vi "read event.vi"() -> ()   [LabVIEW 2016]
uses:
  <vilib>/Instr/_visa.llb/Select Event Type.ctl
  <vilib>/Utility/error.llb/DialogType.ctl
  <vilib>/Instr/_visa.llb/VISA Configure Serial Port (Instr).vi
panel:
  out "error out":errorcluster
  out "recv bytes":u32
  out "Waveform Chart":dbl(graph)
  out "read buffer":string
  in  "VISA resource name":refnum<visa-resource-name>
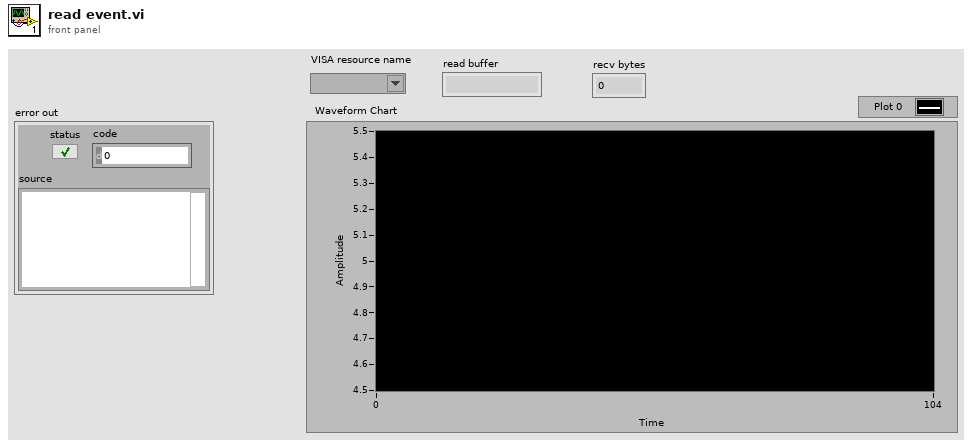
[diagram p1: front panel]
types:
  T1 = typedef "Select Event Type.ctl" = u32
  T2 = typedef "DialogType.ctl" = u16
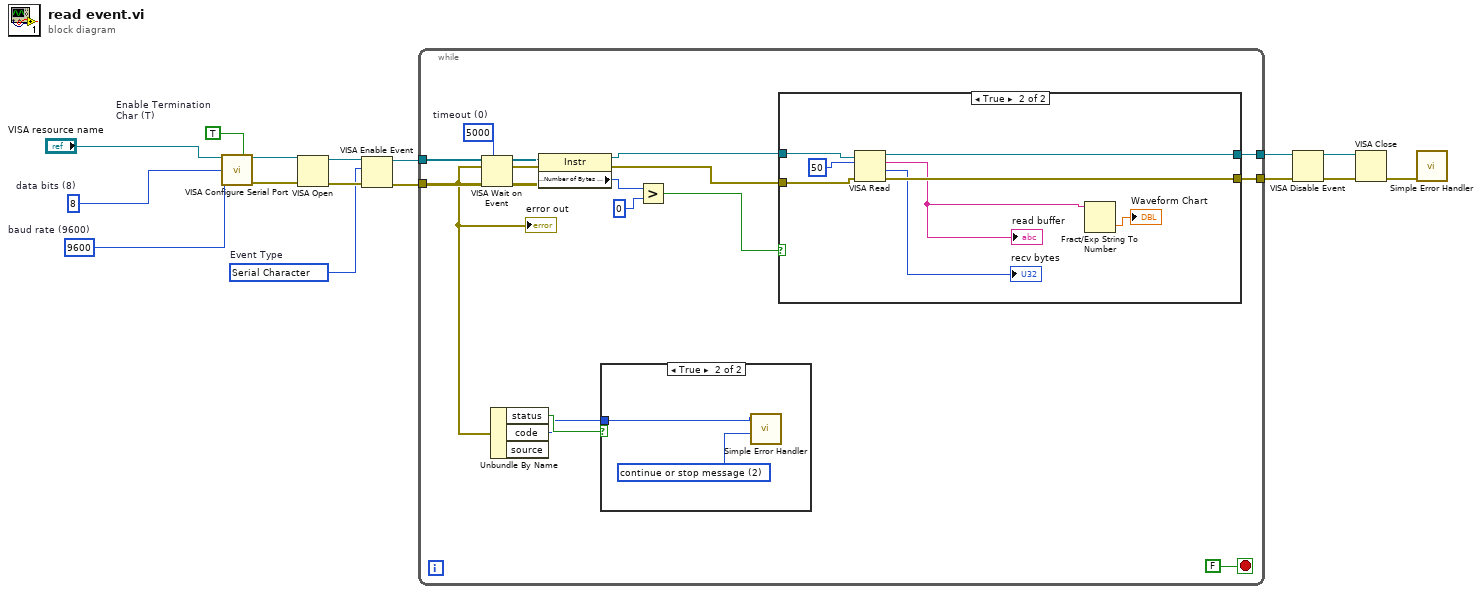
[diagram p0: block diagram]
diagram:
  w4 = u16 8  # data bits (8)
  w5 = TRUE  # Enable Termination Char (T)
  w6 = T1 1073684533 items=["Service Request"=1073684491, "Trigger"=3221168138, "Clear"=1073684493, "VXI Signal"=1073684512, "VXI/VME Interrupt"=3221168161, "VXI/VME Sysfail"=1073684509, "VXI/VME Sysreset"=1073684510, "GPIB CIC"=1073684498, "GPIB Talk"=1073684499, "GPIB Listen"=1073684500, "PXI Interrupt"=1073684514, "Serial Break"=1073684515, "Serial TermChar"=1073684516, "Serial CTS"=1073684521, "Serial DSR"=1073684522, "Serial DCD"=1073684524, "Serial RI"=1073684526, "Serial Character"=1073684533, "USB Interrupt"=1073684535, "All Enabled"=1073709055]  # Event Type
  w15 = u32 9600  # baud rate (9600)
  n1 = call-poly "VISA Configure Serial Port"("VISA resource name"="VISA resource name", "Enable Termination\nChar (T)"=w5, "baud rate (9600)"=w15, "data bits (8)"=w4) -> ("VISA resource name out"=w14:refnum<visa-resource-name>, "error out"=w13:errorcluster)  [unwired: 10 in]
  n2 = VISA Open(error in (no error)=w13, VISA resource name=w14) -> (VISA resource name=w12:refnum<visa-resource-name>, error out=w11:errorcluster)  [unwired: 3 in]
  n3 = VISA Enable Event(8:w11, 10:w6, 11:w12) -> (0:w9:errorcluster, 3:w10:refnum<visa-resource-name>)  [unwired: 1 in]
  n4 = while {
    tunnel: w10 -> [w31]
    tunnel: w9 -> [w30]
    tunnel: [w29] -> w8
    tunnel: [w28] -> w7
    stop <- FALSE stop-if-true
    w21 = u32 5000  # timeout (0)
    n5 = VISA Wait on Event(7:w21, 8:w30, 11:w31) -> (0:w19:errorcluster, 3:w27:refnum<visa-resource-name>)  [unwired: 2 in, 2 out]
    "error out" <- w19
    n6 = Unbundle By Name(w19) -> ("status"=w18:bool, "code"=w17:i32)  [unwired: 1 out]
    n7 = property class="Instr"(reference=w27, error in=w19) -> (reference out=w26:refnum<visa-resource-name>, error out=w22:errorcluster, "Serial Settings:Number of Bytes at Serial Port"=w25:u32)
    n8 = case shown="True" w18 {
      tunnel: w17 -> [_ w33]
      frame False {
      }
      frame True {
        w32 = T2 2 items=["no dialog", "OK message", "continue or stop message", "OK message + warnings", "continue/stop + warnings"] ("type of dialog (OK msg:1)")
        n9 = call <vilib>:"Simple Error Handler.vi"("error code (no error:0)"=w33, "type of dialog (OK msg:1)"=w32) -> ()  [unwired: 3 in, 5 out]
      }
    }
    n10 = Greater?(x=w25, y=u32 0) -> (0:w23:bool)
    n11 = case shown="True" w23 {
      tunnel: [w35 w43] -> w29
      tunnel: [w34 w42] -> w28
      tunnel: w26 -> [w35 w37]
      tunnel: w22 -> [w34 w36]
      frame False {
      }
      frame True {
        n12 = VISA Read(VISA resource name=w37, byte count=u32 50, error in (no error)=w36) -> (VISA resource name out=w43:refnum<visa-resource-name>, read buffer=w40:string, return count=→"recv bytes":u32, error out=w42:errorcluster)
        "read buffer" <- w40
        n13 = Fract/Exp String To Number(string=w40) -> (number=→"Waveform Chart":dbl)  [unwired: 3 in, 1 out]
      }
    }
  }
  n14 = VISA Disable Event(8:w7, 11:w8) -> (0:w3:errorcluster, 3:w2:refnum<visa-resource-name>)  [unwired: 2 in]
  n15 = VISA Close(VISA resource name=w2, error in (no error)=w3) -> (error out=w1:errorcluster)
  n16 = call <vilib>:"Simple Error Handler.vi"("error in (no error)"=w1) -> ()  [unwired: 4 in, 5 out]
